vi "Logging Build Tree.vi"(5 "Entries":T1, 7 "TreeRef":refnum<vi>) -> (3 "TreeRef":refnum<vi>)   [LabVIEW 2012, in "femtoRoboLib.lvlib"]
uses:
  femtoRoboLib.lvlib
  Controls/Log Entry Block.ctl
  Controls/Log Entry.ctl
  Controls/Log Value Type.ctl
  Controls/Log Value Cluster.ctl
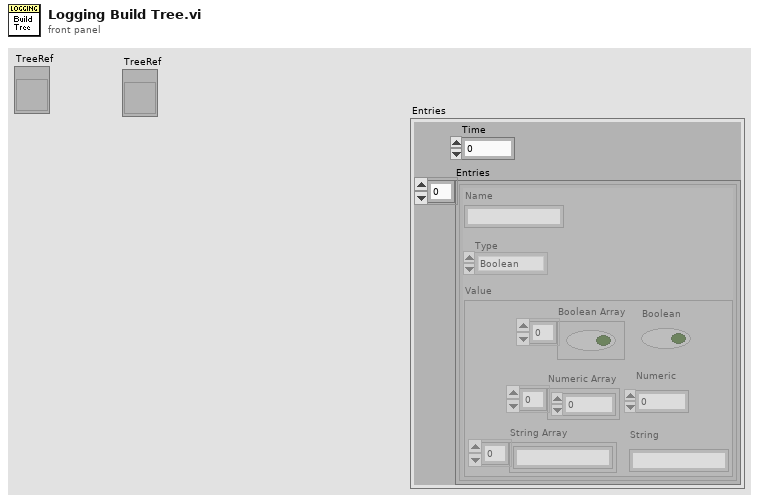
[diagram p1: front panel]
types:
  T1 = typedef "femtoRoboLib.lvlib/Log Entry Block.ctl" = cluster{"Entries":T2[], "Time":u32}
  T2 = typedef "femtoRoboLib.lvlib/Log Entry.ctl" = cluster{"Name":string, "Type":T3, "Value":T4}
  T3 = typedef "femtoRoboLib.lvlib/Log Value Type.ctl" = enum16{"Boolean", "Numeric", "String", "Boolean Array", "Numeric Array", "String Array"}
  T4 = typedef "femtoRoboLib.lvlib/Log Value Cluster.ctl" = cluster{"Boolean Array":bool[], "Boolean":bool, "Numeric Array":dbl[], "Numeric":dbl, "String Array":string[], "String":string}
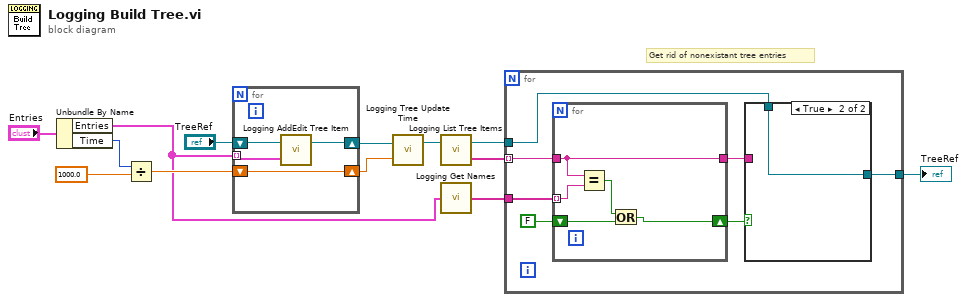
[diagram p0: block diagram]
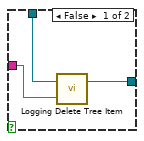
[diagram p2: hidden frame]
diagram:
  # "Get rid of nonexistant tree entries"
  n1 = Unbundle By Name("Entries") -> ("Entries"=w5:T2[], "Time"=w12:u32)
  n2 = Divide(x=w12, y=1000.0) -> (x/y=w8:dbl)
  n3 = for {
    tunnel: w5 -> [w16] mode=indexing
    shift-right: [w15] -> w10
    shift-left: "TreeRef" -> [w17]
    shift-right: [w14] -> w7
    shift-left: w8 -> [w14]
    n4 = call "Logging AddEdit Tree Item.vi"("Log Entry"=w16, "TreeRef"=w17) -> ("TreeRef"=w15:refnum<vi>)  [unwired: 1 in]
  }
  n5 = call "Logging Tree Update Time.vi"("Time"=w7, "TreeRef"=w10) -> ("TreeRef"=w6:refnum<vi>)  [unwired: 1 in]
  n6 = call "Logging List Tree Items.vi"("TreeRef"=w6) -> ("Items"=w4:string[], "TreeRef"=w2:refnum<vi>)  [unwired: 1 in]
  n7 = call "Logging Get Names.vi"("Entries"=w5) -> ("Names"=w3:string[])
  n8 = for {
    tunnel: w4 -> [w22] mode=indexing
    tunnel: w3 -> [w24]
    tunnel: w2 -> [w19]
    tunnel: [w18] -> w1
    n9 = for {
      tunnel: w24 -> [w33] mode=indexing
      shift-right: [w30] -> w21
      shift-left: FALSE -> [w31]
      tunnel: w22 -> [w29]
      tunnel: [w29] -> w20
      n10 = Equal?(x=w29, y=w33) -> (x = y?=w32:bool)
      n11 = Or(x=w32, y=w31) -> (x .or. y?=w30:bool)
    }
    n12 = case shown="True" w21 {
      tunnel: w20 -> [w27 _]
      tunnel: w19 -> [w26 w28]
      tunnel: [w25 w28] -> w18
      frame False {
        n13 = call "Logging Delete Tree Item.vi"("Name"=w27, "TreeRef"=w26) -> ("TreeRef"=w25:refnum<vi>)  [unwired: 1 in]
      }
      frame True {
      }
    }
  }
  "TreeRef" <- w1
